vi "User Event in Device List.vi"(5 "Old List":u16[](array[numeric]), 7 "New List":u16[](array[numeric]), 8 "Error In":errorcluster, 11 "Device List State":T1) -> (0 "Error Out":errorcluster, 3 "Device List State out":T1)   [LabVIEW 2015]
uses:
  Device List State.ctl
  Device/Device.lvclass
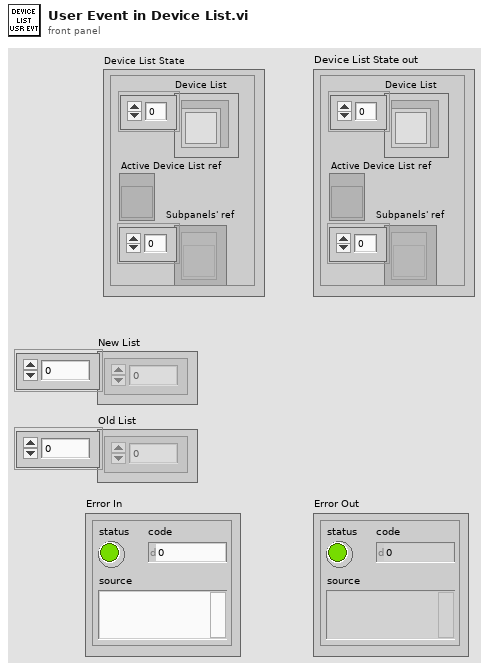
[diagram p1: front panel]
types:
  T1 = typedef "Device List State.ctl" = cluster{"Device List":refnum<class "Device.lvclass">[], "Active Device List ref":refnum<vi>, "Subpanels' ref":refnum<vi>[]}
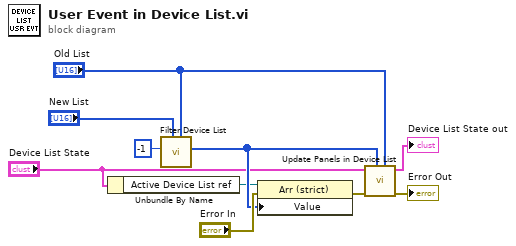
[diagram p0: block diagram]
diagram:
  n1 = Unbundle By Name("Device List State") -> ("Active Device List ref"=w4:refnum<vi>)
  n2 = call "Filter Device List.vi"("Old List"="Old List", "New List"="New List", "Remove object pressed"=-1) -> ("Filtered List"=w9:u16[])  [unwired: 8 in]
  n3 = property class="Arr (strict)"(reference=w4, error in="Error In", "Value"=w9) -> (error out=w8:errorcluster)  [unwired: 1 out]
  n4 = call "Update Panels in Device List.vi"("Old List"="Old List", "New List"=w9, "Error In"=w8, "Device List State"="Device List State") -> ("Error Out"=→"Error Out":errorcluster, "Device List State out"=→"Device List State out":T1)  [unwired: 6 in]
